vi "GetType.vi"(8 "error in (no error)":errorcluster, 11 "Update_Error Msg":refnum<class "Update_Error Msg.lvclass">) -> (0 "error out":errorcluster, 2 "Data Sample":variant, 3 "Update_Error Msg":refnum<class "Update_Error Msg.lvclass">)   [LabVIEW 2015, in "CS++Motor.lvlib" / "Update_Error Msg.lvclass"]
uses:
  Update_Error Msg.lvclass
  Update_Error Msg.lvclass/Update_Error Msg.ctl
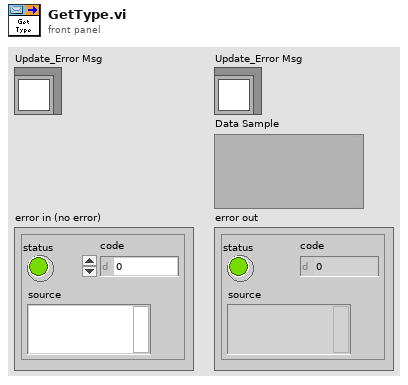
[diagram p1: front panel]
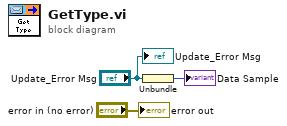
[diagram p0: block diagram]
diagram:
  n1 = Unbundle("Update_Error Msg") -> (→"Data Sample":i8)
  "error out" <- "error in (no error)"
  "Update_Error Msg" <- "Update_Error Msg"
